vi "Caching_Expression_Evaluator_Table.vi"(0 "method":T1, 1 "dt (for table)":dbl, 5 "variable":string, 7 "value in":dbl, 9 "expression/scriptlet":string, 11 "error in (no error)":errorcluster, 12 "steps (for table)":dbl) -> (8 "value out":dbl, 10 "table out":dbl[](array[numeric]), 15 "error out":errorcluster)   [LabVIEW 2013, in "LuaEvaluatorAPI.lvlib"]
doc: "This \"object\" caches variables and parsed expressions for fast evaluation and assignment. It is possible to {set} or {get} a variable, {eval}uate an expression, or evaluate and {assign} an expression to a variable. The {isvalid} method tests whether a variable name is a valid identifier and does not collide with one of the predefined functions or numbers. To set initial values or define custom functions, {execute} a scriptlet.\n\nExpressions and scriptlets can make use Lua's arithmetic operators, the predefined numerical values \"pi\", \"_NaN\", and \"_Inf\", the functions in the math library (sin(), sqrt(), etc.) and the lv library functions for bitwise and other integer operations (andU32(), addI8(), etc.). To promote compact expressions, both sets of functions are available only without their library (\"math.\", \"lv.\") table prefix."
uses:
  LuaEvaluatorAPI.lvlib
  t_Caching_Expression_Evaluator_Methods_Table.ctl
  LuaVIEW1.2.2_full_LV85/luaview/subvis/private/LuaVIEW Push (string).vi
  LuaVIEW1.2.2_full_LV85/luaview/subvis/private/LuaVIEW Push (number).vi
  LuaVIEW1.2.2_full_LV85/luaview/subvis/private/LuaVIEW Pull (number).vi
  LuaVIEW1.2.2_full_LV85/luaview/subvis/private/LuaVIEW Pull (flat data).vi
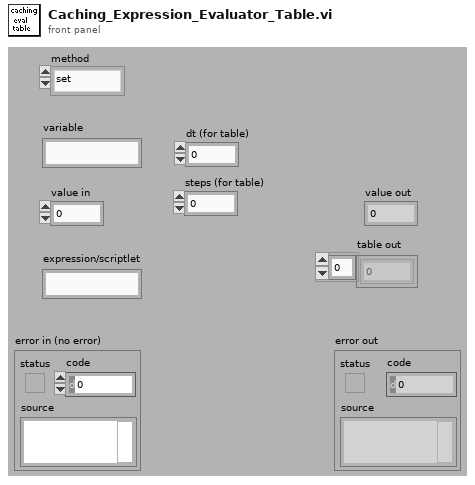
[diagram p1: front panel]
types:
  T1 = typedef "LuaEvaluatorAPI.lvlib/t_Caching_Expression_Evaluator_Methods_Table.ctl" = enum16{"set", "get", "eval", "assign", "isvalid", "execute", "evaltable", "close"}
  T2 = typedef "t_LuaVIEW Reference.ctl" = refnum<k1>
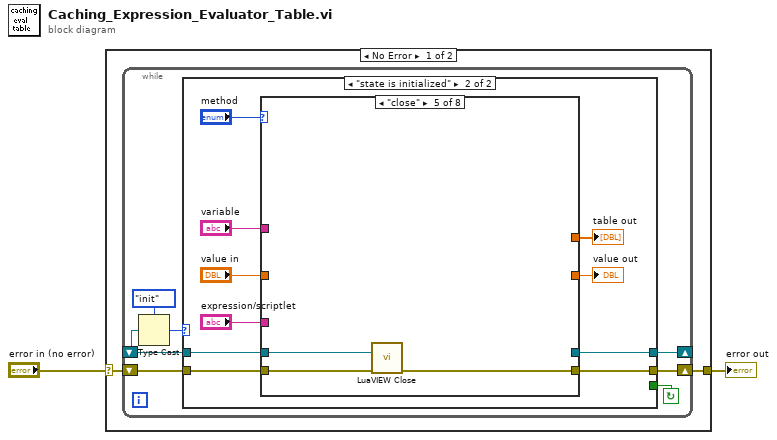
[diagram p0: block diagram]
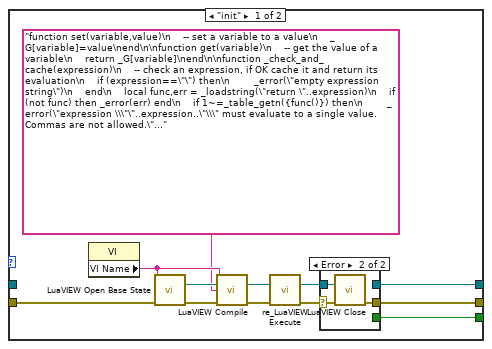
[diagram p2: hidden frame]
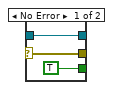
[diagram p3: hidden frame]
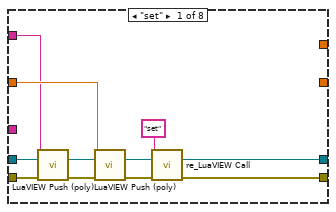
[diagram p4: hidden frame]
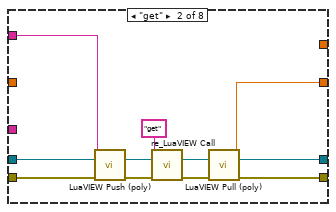
[diagram p5: hidden frame]
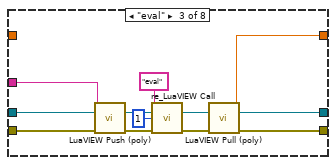
[diagram p6: hidden frame]
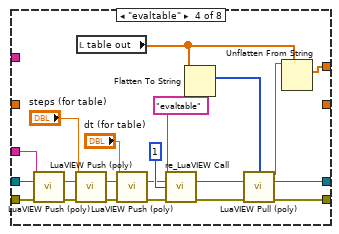
[diagram p7: hidden frame]
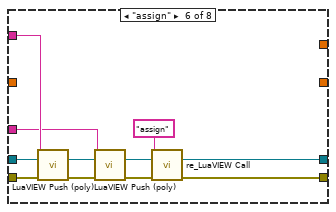
[diagram p8: hidden frame]
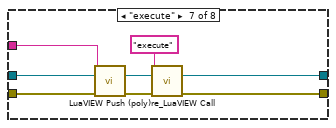
[diagram p9: hidden frame]
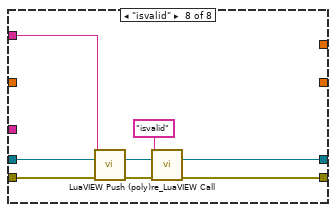
[diagram p10: hidden frame]
diagram:
  n1 = case shown="No Error" "error in (no error)" {
    selector: "error in (no error)" -> [w3 w125]
    tunnel: [w4 w125] -> w1
    frame No Error {
      n2 = while {
        shift-right: [w10] -> _
        shift-left: _ -> [w8]
        shift-right: [w9] -> w4
        shift-left: w3 -> [w11]
        stop <- w5 continue-if-true
        n3 = Type Cast(type=enum32{"init", "state is initialized"}."init", x=w8) -> (*(type *) &x=w6:enum32{"init", "state is initialized"})
        n4 = case shown="\"state is initialized\"" w6 {
          tunnel: w11 -> [w23 w39]
          tunnel: [w13 w36] -> w10
          tunnel: [w14 w37] -> w9
          tunnel: w8 -> [_ w38]
          tunnel: [w12 _] -> w5
          frame "init" {
            n5 = property class="VI"() -> ("VI Name"=w19:string)  [unwired: 2 in, 2 out]
            n6 = call "LuaVIEW Open Base State.vi"("close identifier (none)"=w19, "error in (no error)"=w23) -> ("LuaVIEW reference"=w21:T2, "error out"=w17:errorcluster)  [unwired: 12 out]
            n7 = call "LuaVIEW Compile.vi"("script name"=w19, "LuaVIEW reference in"=w21, "script"="function set(variable,value)\n    -- set a variable to a value\n    _G[variable]=value\nend\n\nfunction get(variable)\n    -- get the value of a variable\n    return _G[variable]\nend\n\nfunction _check_and_cache(expression)\n    -- check an expression, if OK cache it and return its evaluation\n    if (expression==\"\") then\n        _error(\"empty expression string\")\n    end\n    local func,err = _loadstring(\"return \"..expression)\n    if (not func) then _error(err) end\n    if 1~=_table_getn({func()}) then\n        _error(\"expression \\\"\"..expression..\"\\\" must evaluate to a single value. Commas are not allowed.\")\n    end\n    local result=func()\n    if _type(result)~=\"number\" then\n        _error(\"expression \\\"\"..expression..\"\\\" does not evaluate to a number\")\n    end\n    _expression_cache[expression]=func\n    return result\nend\n\nfunction eval(expression)\n    -- evaluate an expression and return its value\n    local func=_expression_cache[expression]\n    if (func) then\n        -- expression already parsed and cached\n        return func()\n    end\n    return _check_and_cache(expression)\nend\n\n-- New code from IBS\nfunction evaltable(expression,steps,TimeStep)\n    -- evaluate an expression and return its value\n    local func=_expression_cache[expression]\n    if (not func) then\n        -- expression not parsed and cached\n        _check_and_cache(expression)\n        func=_expression_cache[expression]\n    end\n    -- expression is now parsed and cached\n    -- now make the desired tabular evaluation\n    \n    local i;\n    local StepsSafe;\n    answer={}\n\n    dt = TimeStep;\n    tMax = (steps+1)*dt;\n    StepsSafe = max(steps,1);\n    for i=0,steps do\n\t       f = i/StepsSafe;\n\t       t = i*dt;\n        answer[i+1] = func()\n    end\n    return answer\nend\n\n\nfunction assign(variable,expression)\n    -- evaluate an expression and assign it to a variable\n    local func=_expression_cache[expression]\n    if (func) then\n        -- expression already parsed and cached\n        _G[variable]=func()\n        return\n    end\n    _G[variable]=_check_and_cache(expression)\nend\n\nfunction execute(statements)\n    -- execute statements, e.g. setting initial variable values\n    -- or defining custom functions\n    local func,err=_loadstring(statements)\n    if (not func) then\n        _error(err)\n    end\n    func()\nend\n\nfunction isvalid(variable)\n    -- check if a variable name is valid for assignment\n    if _name_reserved[variable] then\n        _error(\"\\\"\"..variable..\"\\\" is not a valid variable name: it is reserved for a predefined \".._type(_G[variable]))\n    end\n    if _string_find(variable,\"[^_%w]\") then\n        _error(\"\\\"\"..variable..\"\\\" is not a valid variable name: only underscores and alphanumerical characters are allowed.\")\n    end\n    if (not _loadstring(\"return {\"..variable..\"=42}\")) then\n        _error(\"\\\"\"..variable..\"\\\" is not a valid variable name: leading digits and Lua reserved names are prohibited.\")\n    end    \nend\n\n--start with an empty expression cache\n_expression_cache={}\n\n-- hide functions and tables that do not belong in expressions\n_error=error\n_type=type\n_table_getn=table.getn\n_string_find=string.find\n_loadstring=loadstring\nretain={\nretain=true,\nset=true,\nget=true,\neval=true,\nevaltable=true,\nassign=true,\nexecute=true,\nisvalid=true,\nstring=true,\nmath=true,\n}\nfor k,v in pairs(lv) do\n    if (string.find(k,\"I8\") or string.find(k,\"U8\") or string.find(k,\"I16\") or string.find(k,\"U16\") or string.find(k,\"I32\") or string.find(k,\"U32\")) then\n        _G[k]=v\n        retain[k]=true\n    end\nend\n_name_reserved={}\nfor k,v in pairs(_G) do\n    if _type(k)==\"string\" and not (retain[k] or math[k] or string.sub(k,1,1)==\"_\") then\n        _G[k]=nil\n    else\n        _name_reserved[k]=true\n    end\nend\nmath=nil\n_name_reserved.math=nil\nretain=nil\n_name_reserved.retain=nil\nstring=nil\n_name_reserved.string=nil\n\nf=0\nt=0\ntMax = 0\ndt = 0", "error in (no error)"=w17) -> ("LuaVIEW reference out"=w20:T2, "error out"=w22:errorcluster)  [unwired: 10 out]
            n8 = call "re_LuaVIEW Execute.vi"("LuaVIEW reference in"=w20, "error in (no error)"=w22) -> ("LuaVIEW reference out"=w15:T2, "error out"=w16:errorcluster)  [unwired: 12 out]
            n9 = case shown="Error" w16 {
              selector: w16 -> [w25 w29]
              tunnel: w15 -> [w26 w28]
              tunnel: [w25 w27] -> w14
              tunnel: [w26 _] -> w13
              tunnel: [TRUE _] -> w12
              frame No Error {
              }
              frame Error {
                n10 = call "LuaVIEW Close.vi"("LuaVIEW reference"=w28, "error in (no error)"=w29) -> ("dup error"=w27:errorcluster)  [unwired: 13 out]
              }
            }
          }
          frame "state is initialized" {
            n11 = case shown="\"close\"" "method" {
              tunnel: w39 -> [w47 w51 w63 w87 w97 w105 w112 w119]
              tunnel: w38 -> [w48 w52 w64 w88 w96 w106 w113 w120]
              tunnel: [w40 w61 w73 w94 w95 w98 w110 w117] -> w37
              tunnel: [w41 w56 w68 w91 _ w99 w111 w118] -> w36
              tunnel: "expression/scriptlet" -> [_ _ w65 w89 _ w100 w109 _]
              tunnel: "value in" -> [w43 _ _ _ _ _ _ _]
              tunnel: "variable" -> [w42 w53 _ _ _ w101 _ w121]
              tunnel: [_ w55 w67 _ _ _ _ _] -> w31
              tunnel: [_ _ _ w76 _ _ _ _] -> w30
              frame "set" {
                n12 = call-poly "LuaVIEW Push (poly).vi"("string"=w42, "LuaVIEW reference in"=w48, "error in (no error)"=w47) -> ("LuaVIEW reference out"=w45:T2, "error out"=w46:errorcluster)  [unwired: 11 out]
                n13 = call-poly "LuaVIEW Push (poly).vi"("number"=w43, "LuaVIEW reference in"=w45, "error in (no error)"=w46) -> ("LuaVIEW reference out"=w49:T2, "error out"=w50:errorcluster)  [unwired: 11 out]
                n14 = call "re_LuaVIEW Call.vi"("function name"="set", "LuaVIEW reference in"=w49, "error in (no error)"=w50) -> ("LuaVIEW reference out"=w41:T2, "error out"=w40:errorcluster)  [unwired: 11 out]
              }
              frame "get" {
                n15 = call-poly "LuaVIEW Push (poly).vi"("string"=w53, "LuaVIEW reference in"=w52, "error in (no error)"=w51) -> ("LuaVIEW reference out"=w59:T2, "error out"=w60:errorcluster)  [unwired: 11 out]
                n16 = call "re_LuaVIEW Call.vi"("function name"="get", "LuaVIEW reference in"=w59, "error in (no error)"=w60) -> ("LuaVIEW reference out"=w57:T2, "error out"=w58:errorcluster)  [unwired: 11 out]
                n17 = call-poly "LuaVIEW Pull (poly).vi"("LuaVIEW reference in"=w57, "error in (no error)"=w58) -> ("number"=w55:dbl, "LuaVIEW reference out"=w56:T2, "error out"=w61:errorcluster)  [unwired: 11 out]
              }
              frame "eval" {
                n18 = call-poly "LuaVIEW Push (poly).vi"("string"=w65, "LuaVIEW reference in"=w64, "error in (no error)"=w63) -> ("LuaVIEW reference out"=w71:T2, "error out"=w72:errorcluster)  [unwired: 11 out]
                n19 = call "re_LuaVIEW Call.vi"("function name"="eval", "LuaVIEW reference in"=w71, "required results (no checking needed)"=1, "error in (no error)"=w72) -> ("LuaVIEW reference out"=w69:T2, "error out"=w70:errorcluster)  [unwired: 10 out]
                n20 = call-poly "LuaVIEW Pull (poly).vi"("LuaVIEW reference in"=w69, "error in (no error)"=w70) -> ("number"=w67:dbl, "LuaVIEW reference out"=w68:T2, "error out"=w73:errorcluster)  [unwired: 11 out]
              }
              frame "evaltable" {
                n21 = call-poly "LuaVIEW Push (poly).vi"("string"=w89, "LuaVIEW reference in"=w88, "error in (no error)"=w87) -> ("LuaVIEW reference out"=w85:T2, "error out"=w84:errorcluster)  [unwired: 11 out]
                n22 = call-poly "LuaVIEW Push (poly).vi"("number"="steps (for table)", "LuaVIEW reference in"=w85, "error in (no error)"=w84) -> ("LuaVIEW reference out"=w83:T2, "error out"=w82:errorcluster)  [unwired: 11 out]
                n23 = local read "table out"() -> (w77:dbl[])
                n24 = call-poly "LuaVIEW Push (poly).vi"("number"="dt (for table)", "LuaVIEW reference in"=w83, "error in (no error)"=w82) -> ("LuaVIEW reference out"=w80:T2, "error out"=w81:errorcluster)  [unwired: 11 out]
                n25 = call "re_LuaVIEW Call.vi"("function name"="evaltable", "LuaVIEW reference in"=w80, "required results (no checking needed)"=1, "error in (no error)"=w81) -> ("LuaVIEW reference out"=w92:T2, "error out"=w93:errorcluster)  [unwired: 10 out]
                n26 = Flatten To String(anything=w77) -> (type string=w75:i16[])  [unwired: 1 in, 4 out]
                n27 = call-poly "LuaVIEW Pull (poly).vi"("type descriptor"=w75, "LuaVIEW reference in"=w92, "error in (no error)"=w93) -> ("flat data"=w74:string, "LuaVIEW reference out"=w91:T2, "error out"=w94:errorcluster)  [unwired: 10 out]
                n28 = Unflatten From String(type=w77, binary string=w74) -> (value=w76:dbl[])  [unwired: 1 in, 4 out]
              }
              frame "close" {
                n29 = call "LuaVIEW Close.vi"("LuaVIEW reference"=w96, "error in (no error)"=w97) -> ("dup error"=w95:errorcluster)  [unwired: 13 out]
              }
              frame "assign" {
                n30 = call-poly "LuaVIEW Push (poly).vi"("string"=w101, "LuaVIEW reference in"=w106, "error in (no error)"=w105) -> ("LuaVIEW reference out"=w103:T2, "error out"=w104:errorcluster)  [unwired: 11 out]
                n31 = call-poly "LuaVIEW Push (poly).vi"("string"=w100, "LuaVIEW reference in"=w103, "error in (no error)"=w104) -> ("LuaVIEW reference out"=w107:T2, "error out"=w108:errorcluster)  [unwired: 11 out]
                n32 = call "re_LuaVIEW Call.vi"("function name"="assign", "LuaVIEW reference in"=w107, "error in (no error)"=w108) -> ("LuaVIEW reference out"=w99:T2, "error out"=w98:errorcluster)  [unwired: 11 out]
              }
              frame "execute" {
                n33 = call-poly "LuaVIEW Push (poly).vi"("string"=w109, "LuaVIEW reference in"=w113, "error in (no error)"=w112) -> ("LuaVIEW reference out"=w115:T2, "error out"=w116:errorcluster)  [unwired: 11 out]
                n34 = call "re_LuaVIEW Call.vi"("function name"="execute", "LuaVIEW reference in"=w115, "error in (no error)"=w116) -> ("LuaVIEW reference out"=w111:T2, "error out"=w110:errorcluster)  [unwired: 11 out]
              }
              frame "isvalid" {
                n35 = call-poly "LuaVIEW Push (poly).vi"("string"=w121, "LuaVIEW reference in"=w120, "error in (no error)"=w119) -> ("LuaVIEW reference out"=w123:T2, "error out"=w124:errorcluster)  [unwired: 11 out]
                n36 = call "re_LuaVIEW Call.vi"("function name"="isvalid", "LuaVIEW reference in"=w123, "error in (no error)"=w124) -> ("LuaVIEW reference out"=w118:T2, "error out"=w117:errorcluster)  [unwired: 11 out]
              }
            }
            "value out" <- w31
            "table out" <- w30
          }
        }
      }
    }
    frame Error {
    }
  }
  "error out" <- w1
